vi "Substract axes array subset from axes array.vi"(2 "Axes to query":string[](array[string]), 3 "Axes subset":string[](array[string])) -> (14 "Axes to command":string[](array[string]), 15 "All present?":bool, 16 "Is to command?":bool[](array[boolean]))   [LabVIEW 2020]
doc: "This VI returns only these axes IDs from the Axes to query array which are not \npresent in the Axes subset array. If no axes IDs are returned, All present? is TRUE. Needed by Define axes to command from boolean array.vi."
panel:
  # "This vi returns only these axes IDs from the Axes to query array which are not present in the \nAxes subset array. If no axes IDs are returned, \"All present?\" is TRUE. Is present? returns if Axis\nto query was present in Axes subset or not."
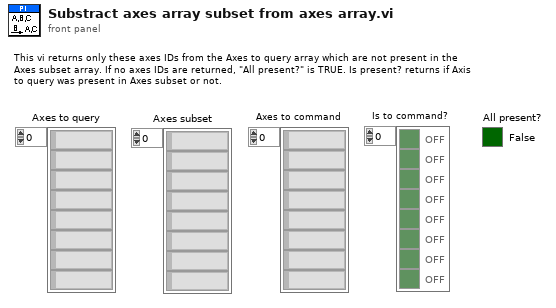
[diagram p1: front panel]
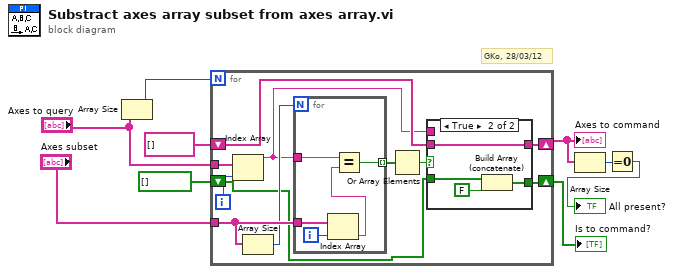
[diagram p0: block diagram]
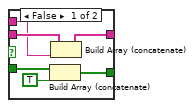
[diagram p2: hidden frame]
diagram:
  # "GKo, 28/03/12"
  n1 = Array Size(array="Axes to query") -> (size(s)=w9:i32)
  n2 = for {
    N: w9 -> [_]
    shift-right: [w14] -> w4
    shift-left: string[] [] -> [w13]
    tunnel: "Axes to query" -> [w20]
    tunnel: "Axes subset" -> [w19]
    shift-right: [w11] -> w1
    shift-left: bool[] [] -> [w10]
    i -> [w17]
    n3 = Index Array(array=w20, index=w17) -> (element=w12:string)
    n4 = Array Size(array=w19) -> (size(s)=w18:i32)
    n5 = for {
      N: w18 -> [_]
      tunnel: w12 -> [w31]
      tunnel: w19 -> [w35]
      tunnel: [w32] -> w16 mode=indexing
      i -> [w34]
      n6 = Index Array(array=w35, index=w34) -> (element=w33:string)
      n7 = Equal?(x=w31, y=w33) -> (x = y?=w32:bool)
    }
    n8 = Or Array Elements(Boolean array=w16) -> (logical OR=w15:bool)
    n9 = case shown="True" w15 {
      tunnel: [w26 w30] -> w14
      tunnel: w13 -> [w25 w30]
      tunnel: w12 -> [w24 _]
      tunnel: [w23 w27] -> w11
      tunnel: w10 -> [w22 w28]
      frame False {
        n10 = Build Array (concatenate)(w22, TRUE) -> (w23:bool[])
        n11 = Build Array (concatenate)(w25, w24) -> (w26:string[])
      }
      frame True {
        n12 = Build Array (concatenate)(w28, FALSE) -> (w27:bool[])
      }
    }
  }
  "Axes to command" <- w4
  "Is to command?" <- w1
  n13 = Array Size(array=w4) -> (size(s)=w5:i32)
  n14 = Equal To 0?(x=w5) -> (x = 0?=→"All present?":bool)
